vi "Insert Into Subpanel.vi"(8 "error in (no error)":errorcluster, 11 "Actor API in":refnum<class "Actor API.lvclass">) -> (0 "error out":errorcluster)   [LabVIEW 2015, in "Actor API.lvclass"]
uses:
  Actor API.lvclass
  <vilib>/event_ctls.llb/usereventprio.ctl
  Messaging/Message/Message.lvclass/Message.ctl
  Messaging/Message/Message.lvclass
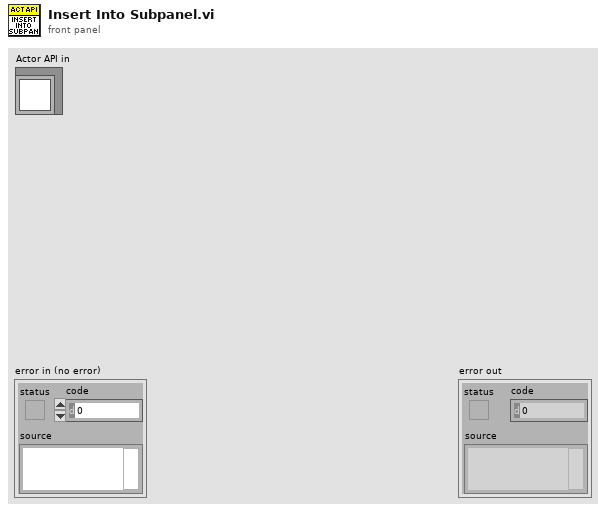
[diagram p1: front panel]
types:
  T1 = typedef "usereventprio.ctl" = enum32{"high priority", "normal priority"}
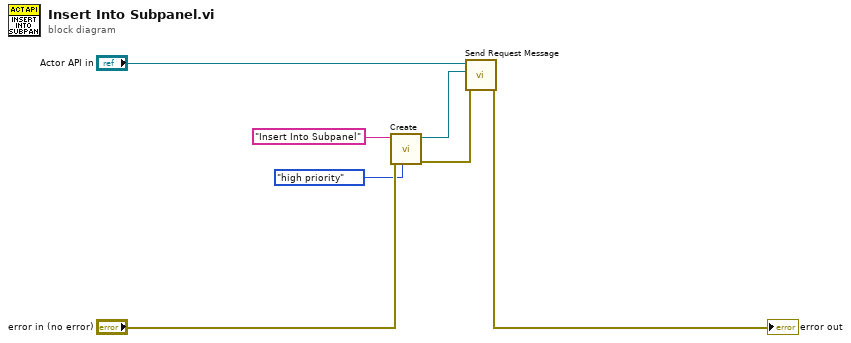
[diagram p0: block diagram]
diagram:
  n1 = call "Create.vi"("Priority (normal)"=usereventprio."high priority", "error in (no error)"="error in (no error)", "Name"="Insert Into Subpanel" ("format string")) -> ("error out"=w3:errorcluster, "Message out"=w2:refnum<class "Message.lvclass">)  [unwired: 7 in]
  n2 = call-dynamic "Send Request Message.vi"("error in (no error)"=w3, "Message"=w2, "Actor API in"="Actor API in") -> ("error out"=→"error out":errorcluster)  [unwired: 8 in]
